vi "Trim Whitespace [Inlined].vi"(0 "string":string, 1 "location (both)":T1 items=["both", "start of string", "end of string"]) -> (2 "trimmed string":string)   [LabVIEW 2020]
doc: "Removes all ASCII white space (spaces, tabs, carriage returns, and linefeeds) from the beginning, end, or both ends of <B>string</B>. The Trim Whitespace VI does not remove double byte characters."
uses:
  <vilib>/Utility/error.llb/whitespace.ctl
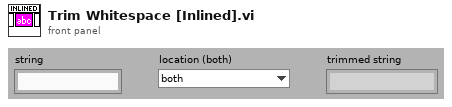
[diagram p1: front panel]
types:
  T1 = typedef "whitespace.ctl" = u16
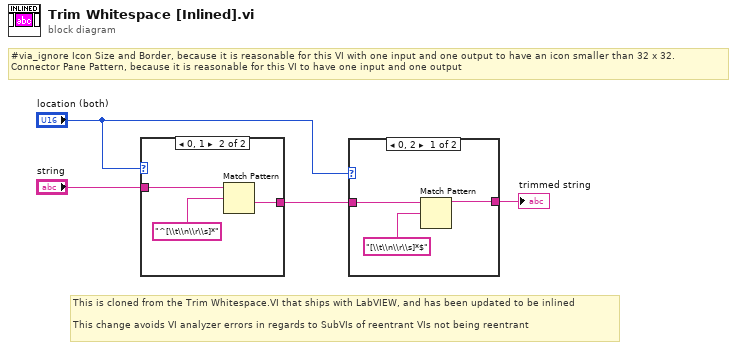
[diagram p0: block diagram]
diagram:
  # "#via_ignore Icon Size and Border, because it is reasonable for this VI with one input and one output to have an icon smaller than 32 x 32.\nConnector Pane Pattern, because it is reasonable for this VI to have one input and one output"
  # "This is cloned from the Trim Whitespace.VI that ships with LabVIEW, and has been updated to be inlined\n\nThis change avoids VI analyzer errors in regards to SubVIs of reentrant VIs not being reentrant"
  n1 = case shown="0, 1" "location (both)" {
    tunnel: [w5 w8] -> w3
    tunnel: "string" -> [w5 w6]
    frame Default {
    }
    frame 0, 1 {
      n2 = Match Pattern(string=w6, regular expression="^[\\t\\n\\r\\s]*") -> (after substring=w8:string)  [unwired: 1 in, 3 out]
    }
  }
  n3 = case shown="0, 2" "location (both)" {
    tunnel: [w11 w12] -> w4
    tunnel: w3 -> [w10 w12]
    frame 0, 2 {
      n4 = Match Pattern(string=w10, regular expression="[\\t\\n\\r\\s]*$") -> (before substring=w11:string)  [unwired: 1 in, 3 out]
    }
    frame Default {
    }
  }
  "trimmed string" <- w4
